vi "open.vi"(0 "M1M3Settings in":refnum<class "M1M3Settings.lvclass">, 11 "error in (no error)":errorcluster) -> (4 "M1M3Settings out":refnum<class "M1M3Settings.lvclass">, 6 "SelectedSet":string, 8 "SelectedVersion":string, 10 "Canceled":bool, 15 "error out":errorcluster)   [LabVIEW 2016, in "M1M3Settings.lvclass"]
uses:
  M1M3Settings.lvclass
  D:/Code/ts_M1M3Support/Settings/Settings/Setting.lvclass
  Settings/Setting.lvclass/Setting.ctl
  Settings/Setting.lvclass
panel:
  in  "Create New":bool
  in  "Cancel":bool
  in  "Edit Selected":bool
  in  "Available Settings":i32(listbox)
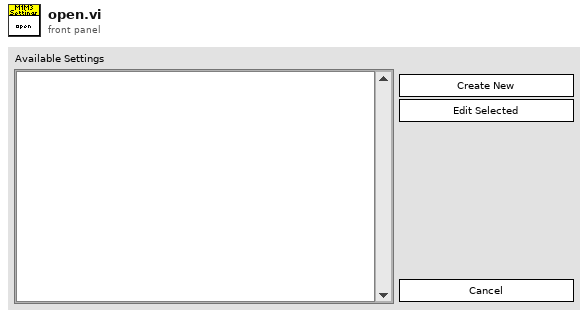
[diagram p1: front panel]
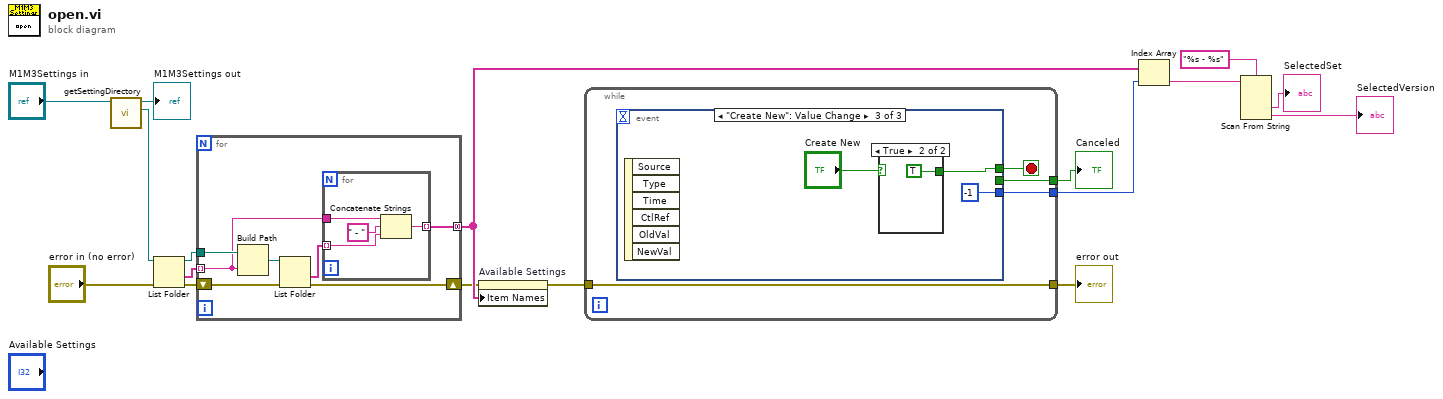
[diagram p0: block diagram]
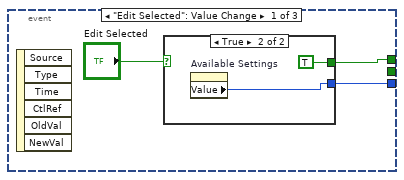
[diagram p2: hidden frame]
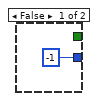
[diagram p3: hidden frame]
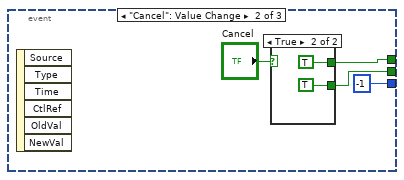
[diagram p4: hidden frame]
diagram:
  n1 = call "getSettingDirectory.vi"("BaseSetting in"="M1M3Settings in") -> ("SettingDirectory"=w11:path, "BaseSetting out"=→"M1M3Settings out":refnum<class "M1M3Settings.lvclass">)  [unwired: 9 in]
  n2 = List Folder(path=w11, error in="error in (no error)") -> (path out=w9:path, folder names=w10:string[], error out=w6:errorcluster)  [unwired: 2 in, 1 out]
  n3 = for {
    tunnel: w10 -> [w21] mode=indexing
    tunnel: w9 -> [w24]
    tunnel: [w20] -> w8 mode=concatenating
    shift-right: [w18] -> w5
    shift-left: w6 -> [w19]
    n4 = Build Path(base path=w24, name or relative path=w21) -> (appended path=w23:path)
    n5 = List Folder(path=w23, error in=w19) -> (folder names=w22:string[], error out=w18:errorcluster)  [unwired: 2 in, 2 out]
    n6 = for {
      tunnel: w22 -> [w27] mode=indexing
      tunnel: w21 -> [w28]
      tunnel: [w25] -> w20 mode=indexing
      n7 = Concatenate Strings(w28, " - " ("string"), w27) -> (w25:string)
    }
  }
  n8 = property on="Available Settings" class="LstBox (strict)"(error in=w5, "Item Names"=w8) -> (error out=w14:errorcluster)  [unwired: 1 in, 1 out]
  n9 = while {
    tunnel: [w31] -> w12
    tunnel: [w30] -> w16
    tunnel: [w29] -> w15
    tunnel: w14 -> [w29]
    stop <- w32 stop-if-true
    n10 = event shown="[2] \"Create New\": Value Change" {
      selector: _ -> [_ _ _]
      dyn-events: _ -> [_ _ _]
      timeout: _ -> [_ _ _]
      tunnel: [w34 w41 w45] -> w32
      tunnel: [_ w40 _] -> w31
      tunnel: [w33 -1 ("Value") -1 ("Value")] -> w30
      event "Edit Selected": Value Change {
        n11 = event-data() -> ()  [unwired: 1 in, 6 out]
        n12 = case shown="True" "Edit Selected" {
          tunnel: [_ TRUE] -> w34
          tunnel: [-1 ("Value") w37] -> w33
          frame False {
          }
          frame True {
            n13 = property on="Available Settings" class="LstBox (strict)"() -> ("Value"=w37:i32)  [unwired: 2 in, 2 out]
          }
        }
      }
      event "Cancel": Value Change {
        n14 = event-data() -> ()  [unwired: 1 in, 6 out]
        n15 = case shown="True" "Cancel" {
          tunnel: [_ TRUE] -> w41
          tunnel: [_ TRUE] -> w40
          frame False {
          }
          frame True {
          }
        }
      }
      event "Create New": Value Change {
        n16 = event-data() -> ()  [unwired: 1 in, 6 out]
        n17 = case shown="True" "Create New" {
          tunnel: [_ TRUE] -> w45
          frame False {
          }
          frame True {
          }
        }
      }
    }
  }
  "error out" <- w15
  "Canceled" <- w12
  n18 = Index Array(array=w8, index=w16) -> (element=w3:string)
  n19 = Scan From String(format string="%s - %s", input string=w3) -> (output 1=→"SelectedSet":string, output 2=→"SelectedVersion":string)  [unwired: 4 in, 3 out]
